vi "Set myRIO Image.vi"() -> ()   [LabVIEW 2014]
uses:
  <vilib>/nisyscfg/Set System Image (File).vi
  <vilib>/nisyscfg/nisyscfg.lvlib
panel:
  in  "Source File":path=path "C:/Users/blueuser/Desktop/Robo Sim Berkley/cpsgrader-release-0.4/Version 2/iRobot Remote Control.zip"
  in  "Session in":refnum<k21>
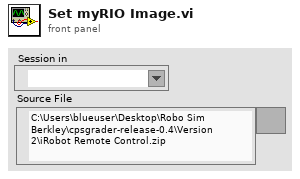
[diagram p1: front panel]
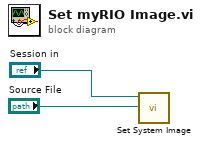
[diagram p0: block diagram]
diagram:
  n1 = call-poly <vilib>:"Set System Image.vi"("Source File"="Source File", "Session in"="Session in") -> ()  [unwired: 8 in, 2 out]
